vi "ARI Function.vi"() -> ()   [LabVIEW 2014]
panel:
  out "Motor Value":dbl
  out "Is Below":bool
  out "Is Above":bool
  in  "stop":bool
  out "coerced(x)":dbl
  out "In Range?":bool
  in  "Input":dbl(slide) scale=0.0..20.0
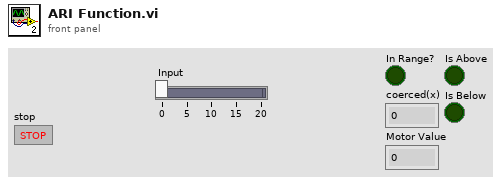
[diagram p1: front panel]
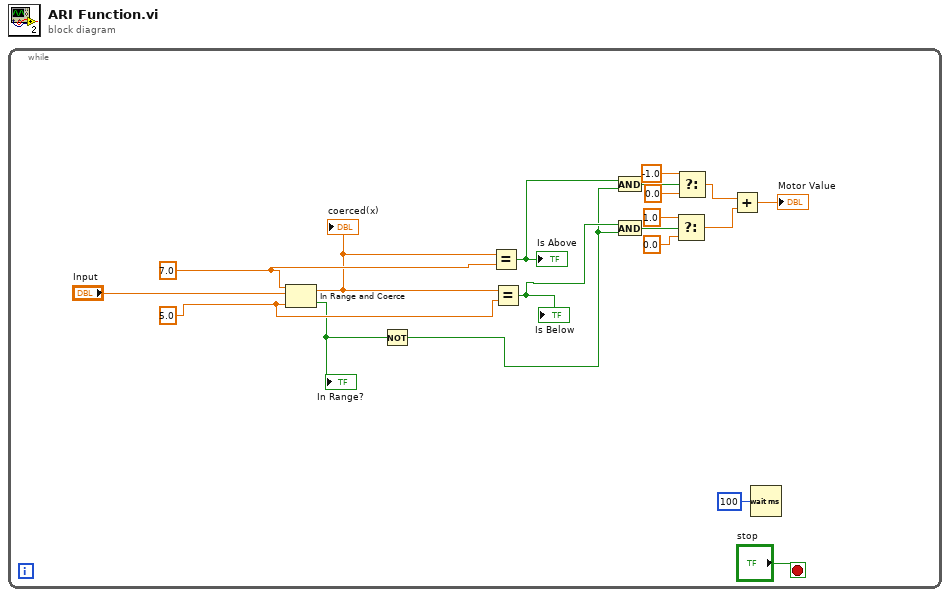
[diagram p0: block diagram]
diagram:
  n1 = while {
    stop <- "stop" stop-if-true
    w15 = 5.0 ("upper limit")
    w16 = 7.0 ("upper limit")
    n2 = In Range and Coerce(upper limit=w16, x="Input", lower limit=w15) -> (coerced(x)=w14:dbl, In Range?=w11:bool)
    "In Range?" <- w11
    "coerced(x)" <- w14
    n3 = Not(x=w11) -> (.not. x?=w8:bool)
    n4 = Equal?(x=w14, y=w16) -> (x = y?=w12:bool)
    "Is Above" <- w12
    n5 = Equal?(x=w14, y=w15) -> (x = y?=w13:bool)
    "Is Below" <- w13
    n6 = And(x=w12, y=w8) -> (x .and. y?=w10:bool)
    n7 = And(x=w13, y=w8) -> (x .and. y?=w9:bool)
    n8 = Select(t=1.0, s=w9, f=0.0) -> (s? t:f=w2:dbl)
    n9 = Select(t=-1.0, s=w10, f=0.0) -> (s? t:f=w3:dbl)
    n10 = Add(x=w3, y=w2) -> (x+y=→"Motor Value":dbl)
    n11 = Wait (ms)(milliseconds to wait=u32 100) -> ()  [unwired: 1 out]
  }
